vi "32intArray_to_Bytes.vi"(11 "Postition to Be Set":i32[](array[numeric])) -> (1 "result":i32, 2 "Array2":u8[](array[numeric]), 3 "Array1":u8[](array[numeric]))   [LabVIEW 2017]
panel:
  in  "start byte":u8=2
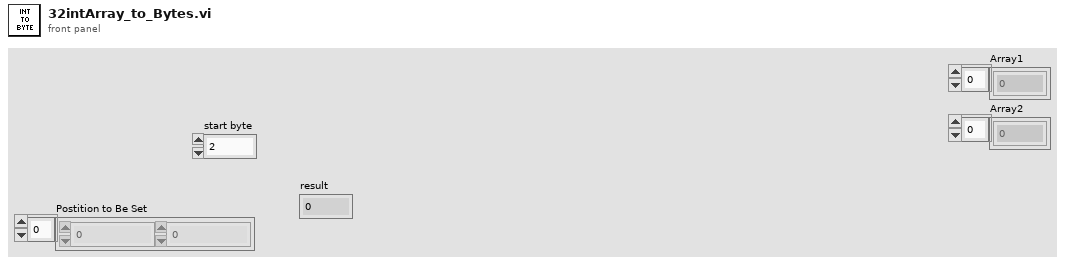
[diagram p1: front panel]
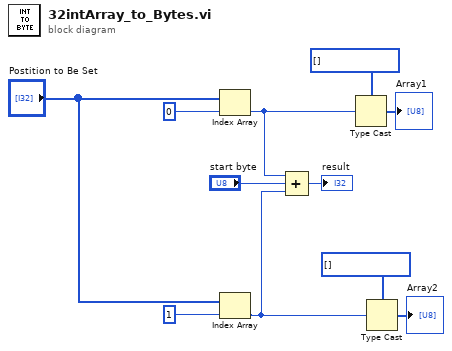
[diagram p0: block diagram]
diagram:
  n1 = Index Array(array="Postition to Be Set", index=0) -> (element=w6:i32)
  n2 = Index Array(array="Postition to Be Set", index=1) -> (element=w5:i32)
  n3 = Compound Arithmetic op=ADD(w6, "start byte", w5) -> (→"result":i32)
  n4 = Type Cast(type=u8[] [], x=w6) -> (*(type *) &x=→"Array1":u8[])
  n5 = Type Cast(type=u8[] [], x=w5) -> (*(type *) &x=→"Array2":u8[])
